vi "Write String.vi"(8 "error in (no error)":errorcluster, 10 "String":string, 11 "class string child in":refnum<class "Child.lvclass">) -> (0 "error out":errorcluster, 3 "class string child out":refnum<class "Child.lvclass">)   [LabVIEW 2023, in "Child.lvclass"]
doc: "Sets the string data for Child.ctl."
uses:
  Child.lvclass
  Child.lvclass/Child.ctl
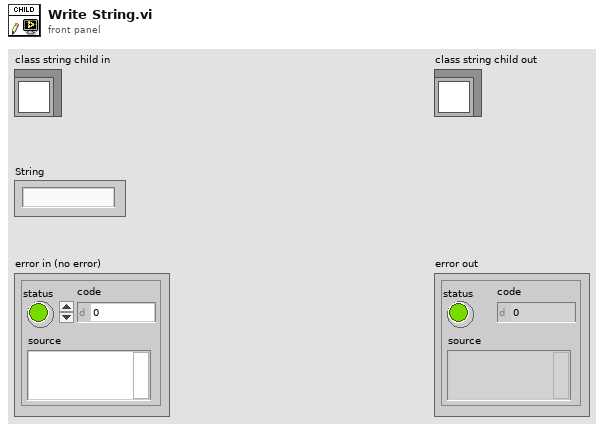
[diagram p1: front panel]
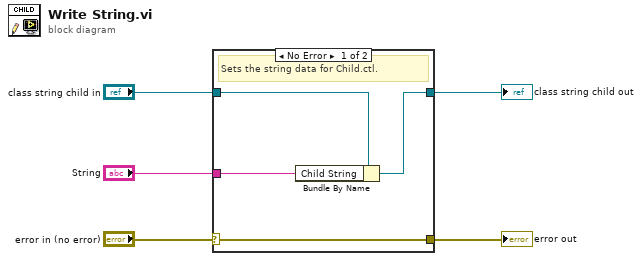
[diagram p0: block diagram]
diagram:
  n1 = case shown="No Error" "error in (no error)" {
    selector: "error in (no error)" -> [w9 w10]
    tunnel: [w9 w10] -> w4
    tunnel: [w8 w11] -> w2
    tunnel: "class string child in" -> [w6 w11]
    tunnel: "String" -> [w7 _]
    frame No Error {
      # "Sets the string data for Child.ctl."
      n2 = Bundle By Name(cluster=w6, "Child String"=w7) -> (w8:refnum<class "Child.lvclass">)
    }
    frame Error {
    }
  }
  "error out" <- w4
  "class string child out" <- w2
